vi "CODMn报警信息转换.vi"(11 "报警簇":T1) -> (1 "code":u64, 2 "CODMN报警信息备注":string, 3 "CODMN报警信息":string)   [LabVIEW 2016, in "斯坦道CODMn.lvlib"]
uses:
  Alarm interface/Alarm interface.lvlib
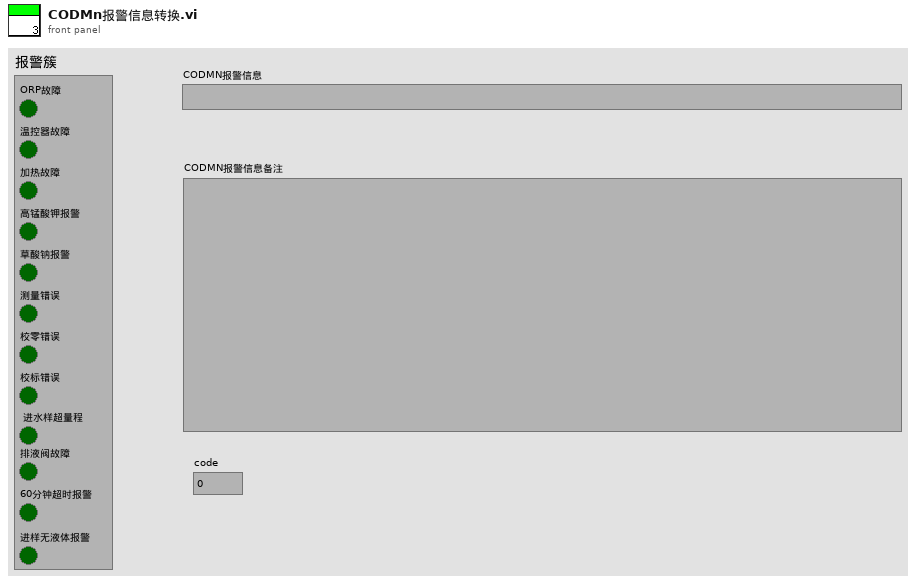
[diagram p1: front panel]
types:
  T1 = cluster{"ORP故障":bool, "温控器故障":bool, "加热故障":bool, "高锰酸钾报警":bool, "草酸钠报警":bool, "测量错误":bool, "校零错误":bool, "校标错误":bool, " 进水样超量程":bool, "排液阀故障":bool, "60分钟超时报警":bool, "进样无液体报警":bool}
  T2 = cluster{"module name":string, "moduleid":i32, "sysid":i32, "content":string, "analysis":string}
  T3 = enum16{"营养盐", "V2CODMn", "新CODMn", "动力环境", "质控单元", "采配水", "其他"}
  T4 = cluster{"modid":i32, "sysid":i32, "content":string, "故障详情":string}
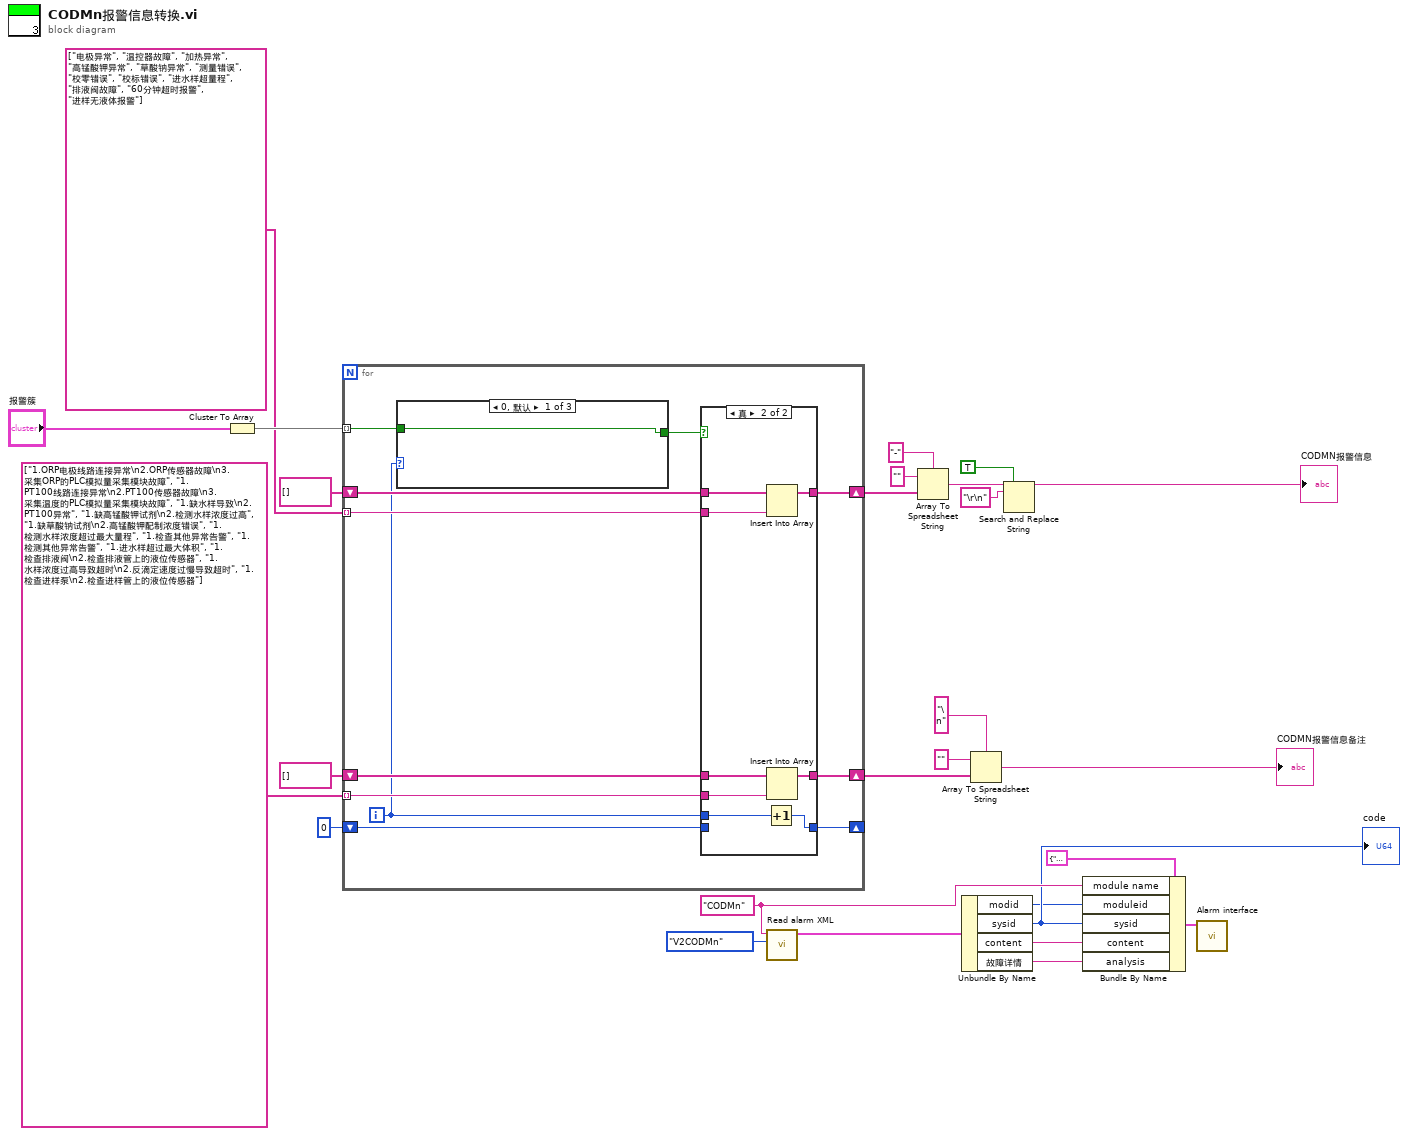
[diagram p0: block diagram]
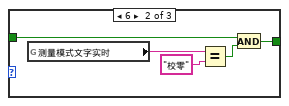
[diagram p2: hidden frame]
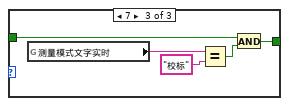
[diagram p3: hidden frame]
diagram:
  w8 = "CODMn" ("模块名称")
  n1 = Cluster To Array(cluster="报警簇") -> (array=w20:bool[])
  n2 = for {
    tunnel: w20 -> [w38] mode=indexing
    shift-right: [w34] -> w15
    shift-left: string[] [] -> [w36]
    tunnel: string[] ["电极异常", "温控器故障", "加热异常", "高锰酸钾异常", "草酸钠异常", "测量错误", "校零错误", "校标错误", "进水样超量程", "排液阀故障", "60分钟超时报警", "进样无液体报警"] -> [w35] mode=indexing
    shift-right: [w31] -> w12
    shift-left: string[] [] -> [w33]
    tunnel: string[] ["1.ORP电极线路连接异常\n2.ORP传感器故障\n3.采集ORP的PLC模拟量采集模块故障", "1.PT100线路连接异常\n2.PT100传感器故障\n3.采集温度的PLC模拟量采集模块故障", "1.缺水样导致\n2.PT100异常", "1.缺高锰酸钾试剂\n2.检测水样浓度过高", "1.缺草酸钠试剂\n2.高锰酸钾配制浓度错误", "1.检测水样浓度超过最大量程", "1.检查其他异常告警", "1.检测其他异常告警", "1.进水样超过最大体积", "1.检查排液阀\n2.检查排液管上的液位传感器", "1.水样浓度过高导致超时\n2.反滴定速度过慢导致超时", "1.检查进样泵\n2.检查进样管上的液位传感器"] -> [w32] mode=indexing
    shift-right: [w29] -> _
    shift-left: 0 -> [w28]
    i -> [w30]
    n3 = case shown="0, 默认" w30 {
      tunnel: w38 -> [w39 w41 w46]
      tunnel: [w39 w40 w45] -> w37
      frame 0, Default {
      }
      frame 6 {
        n4 = global read "COD测量模式全局.vi" "测量模式文字实时"() -> (w43:string)
        n5 = Equal?(x=w43, y="校零" ("测量模式")) -> (x = y?=w42:bool)
        n6 = And(x=w41, y=w42) -> (x .and. y?=w40:bool)
      }
      frame 7 {
        n7 = global read "COD测量模式全局.vi" "测量模式文字实时"() -> (w48:string)
        n8 = Equal?(x=w48, y="校标" ("测量模式")) -> (x = y?=w47:bool)
        n9 = And(x=w46, y=w47) -> (x .and. y?=w45:bool)
      }
    }
    n10 = case shown="真" w37 {
      tunnel: w36 -> [w52 w60]
      tunnel: w35 -> [_ w59]
      tunnel: [w52 w58] -> w34
      tunnel: w33 -> [w51 w57]
      tunnel: w32 -> [_ w56]
      tunnel: [w51 w55] -> w31
      tunnel: w30 -> [_ w54]
      tunnel: [w50 w53] -> w29
      tunnel: w28 -> [w50 _]
      frame False {
      }
      frame True {
        n11 = Increment(x=w54) -> (x+1=w53:i32)
        n12 = Insert Into Array(array=w60, new element=w59) -> (w58:string[])  [unwired: 1 in]
        n13 = Insert Into Array(array=w57, new element=w56) -> (w55:string[])  [unwired: 1 in]
      }
    }
  }
  n14 = call "Read alarm XML.vi"("模块常量"=T3."V2CODMn", "模块名称"=w8) -> ("报警"=w9:T4)  [unwired: 9 in]
  n15 = Array To Spreadsheet String(delimiter (Tab)="-" ("分隔符(Tab)"), array=w15, 3:"" ("格式字符串")) -> (spreadsheet string=w23:string)
  n16 = Unbundle By Name(w9) -> ("modid"=w3:i32, "sysid"=w6:i32, "content"=w2:string, "故障详情"=w1:string)
  "code" <- w6
  n17 = Array To Spreadsheet String(delimiter (Tab)="\n" ("分隔符(Tab)"), array=w12, 3:"" ("格式字符串")) -> (spreadsheet string=→"CODMN报警信息备注":string)
  n18 = Search and Replace String(replace all?=TRUE ("替换全部？(F)"), input string=w23, search string="\r\n" ("搜索字符串")) -> (result string=→"CODMN报警信息":string)  [unwired: 5 in, 3 out]
  n19 = Bundle By Name(cluster=T2 {"module name"="", "moduleid"=0, "sysid"=0, "content"="", "analysis"=""} ("簇"), "module name"=w8, "moduleid"=w3, "sysid"=w6, "content"=w2, "analysis"=w1) -> (w4:T2)
  n20 = call "Alarm interface.vi"("簇"=w4) -> ()  [unwired: 10 in, 1 out]
